vi "runEditor.vi"(8 "error in (no error)":errorcluster, 9 "deviceDataBase":refnum<class "deviceDataBase.lvclass">, 10 "ScriptEdEvents":refnum<class "ScriptEdEvents.lvclass">, 11 "ScriptEditorV2 in":refnum<class "ScriptEditorV2.lvclass">) -> (0 "error out":errorcluster, 3 "ScriptEditorV2 out":refnum<class "ScriptEditorV2.lvclass">)   [LabVIEW 2011, in "Views.lvlib" / "ScriptEditor.lvlib" / "ScriptEditorV2.lvclass"]
doc: "ScriptEditorV2 Run.\n\nlaunches Script editor, which allows users to manipulate scripts."
uses:
  ScriptEditorV2.lvclass
  ScriptEdEvents/ScriptEdEvents.lvclass
  Tools/DatabaseHelpers/DbConnection/DeviceDataBase/deviceDataBase.lvclass
  Tools/Scripting/ScriptingEvent/ScriptEventList/ScriptEventList.lvclass
  ScriptEditorV2.lvclass/ScriptEditorV2.ctl
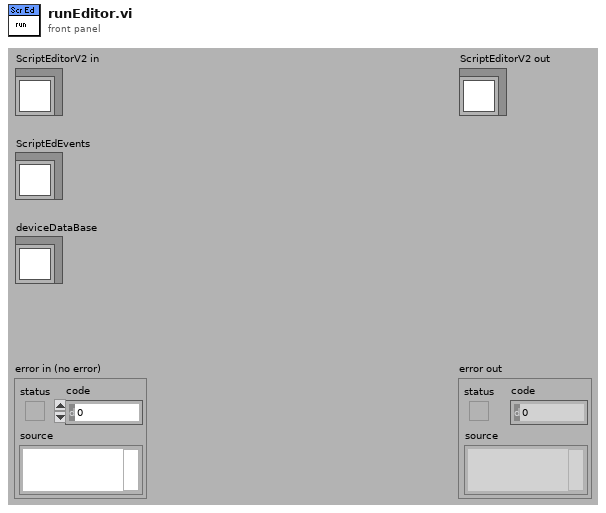
[diagram p1: front panel]
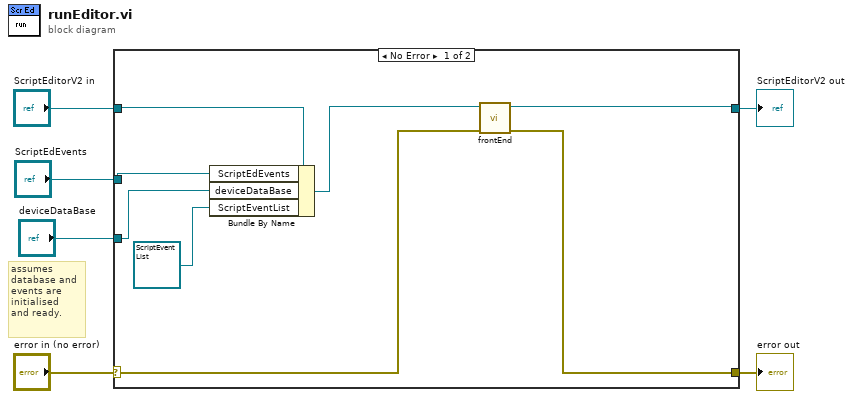
[diagram p0: block diagram]
diagram:
  # "assumes\ndatabase and \nevents are\ninitialised\nand ready."
  n1 = case shown="No Error" "error in (no error)" {
    selector: "error in (no error)" -> [w9 w16]
    tunnel: [w7 w16] -> w5
    tunnel: [w8 w15] -> w3
    tunnel: "ScriptEditorV2 in" -> [w13 w15]
    tunnel: "ScriptEdEvents" -> [w14 _]
    tunnel: "deviceDataBase" -> [w11 _]
    frame No Error {
      n2 = Bundle By Name(cluster=w13, "ScriptEdEvents"=w14, "deviceDataBase"=w11, "ScriptEventList"=refnum<class "ScriptEventList.lvclass"> refnum ("Tools.lvlib:Scripting.lvlib:ScriptEventList.lvclass")) -> (w10:refnum<class "ScriptEditorV2.lvclass">)
      n3 = call "frontEnd.vi"("error in (no error)"=w9, "ScriptEditorV2 in"=w10) -> ("error out"=w7:errorcluster, "ScriptEditorV2 out"=w8:refnum<class "ScriptEditorV2.lvclass">)  [unwired: 8 in]
    }
    frame Error {
    }
  }
  "error out" <- w5
  "ScriptEditorV2 out" <- w3
